vi "设置预设电源波形.vi"(10 "一炮最长运行时间点（ms)":dbl, 11 "预设波形数组":dbl[][](array[numeric])) -> (1 "波形解析正确":bool, 2 "XY Graph":cluster{"xi used":dbl[], "yi":dbl[]}(graph), 3 "插值后输出波形幅值":dbl[](array[numeric]))   [LabVIEW 2018]
panel:
  # "第一列代表时间，第二列代表幅值"
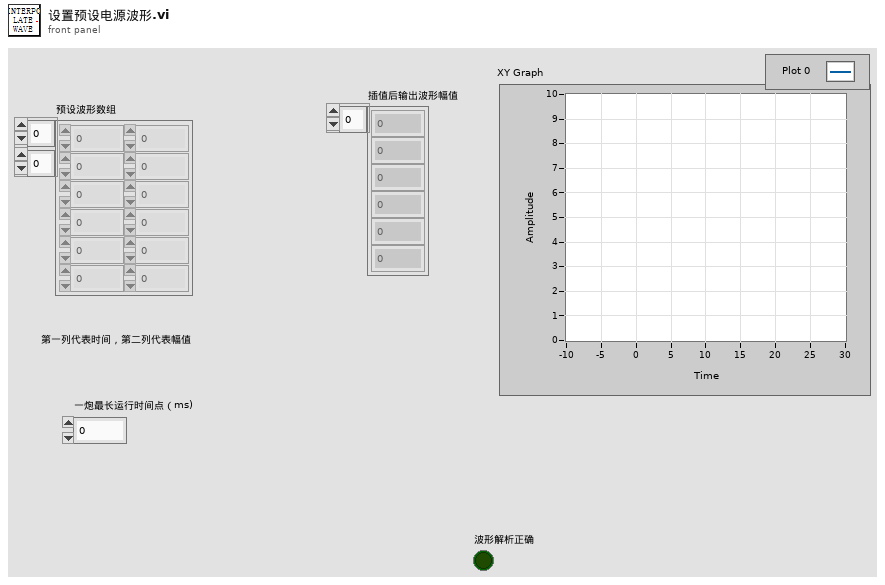
[diagram p1: front panel]
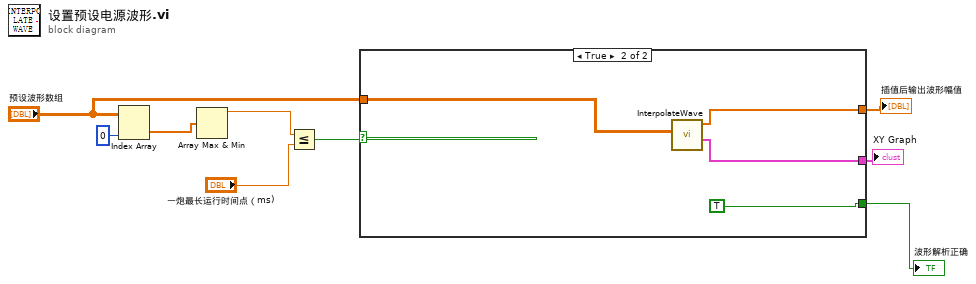
[diagram p0: block diagram]
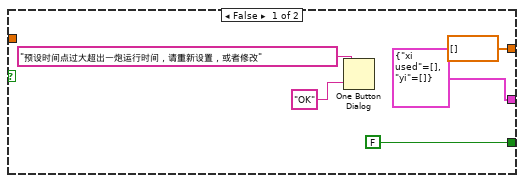
[diagram p2: hidden frame]
diagram:
  n1 = Index Array(array="预设波形数组", index (col)=0 ("disabled index (col)")) -> (element=w8:dbl[])  [unwired: 1 in]
  n2 = Array Max & Min(array=w8) -> (max value=w7:dbl)  [unwired: 3 out]
  n3 = Less Or Equal?(x=w7, y="一炮最长运行时间点（ms)") -> (x <= y?=w5:bool)
  n4 = case shown="True" w5 {
    tunnel: "预设波形数组" -> [_ w18]
    tunnel: [dbl[] [] ("插值后输出波形幅值") w17] -> w3
    tunnel: [cluster{"xi used":dbl[], "yi":dbl[]} {"xi used"=[], "yi"=[]} ("XY Graph") w16] -> w2
    tunnel: [FALSE TRUE] -> w1
    frame False {
      n5 = One Button Dialog(message="预设时间点过大超出一炮运行时间，请重新设置，或者修改", button name ("OK")="OK") -> ()  [unwired: 1 out]
    }
    frame True {
      n6 = call "InterpolateWave.vi"("输出波形预设"=w18) -> ("XY Graph"=w16:cluster{"xi used":dbl[], "yi":dbl[]}, "插值后输出波形幅值"=w17:dbl[])  [unwired: 6 in, 1 out]
    }
  }
  "插值后输出波形幅值" <- w3
  "XY Graph" <- w2
  "波形解析正确" <- w1
